vi "subVI_read_write_ADC_DAC.vi"(7 "CH":bool[](array[boolean])=[FALSE, FALSE, TRUE, FALSE, FALSE, TRUE, FALSE, FALSE, FALSE, FALSE, FALSE, FALSE, FALSE, FALSE, FALSE, FALSE], 8 "DAC2":bool[](array[boolean]), 9 "DAC1":bool[](array[boolean]), 10 "error in":errorcluster, 11 "FPGA VI Reference In":refnum<k20>) -> (0 "FPGA VI Reference Out":refnum<k20>, 1 "i":dbl, 2 "GAIN":i16, 3 "UNI":i16, 4 "error out":errorcluster)   [LabVIEW 2018]
uses:
  <vilib>/Utility/error.llb/Error Cluster From Error Code.vi
  <vilib>/rvi/errors/niLvFpgaAdjustHostInterfaceError.vi
  <vilib>/rvi/interface/nirviReadWriteControl/nirviReadWriteControl.xnode
  NiFpgaLv.dll
  <vilib>/rvi/interface/Simulation/niFpgaSimulationCallBeginRW.vi
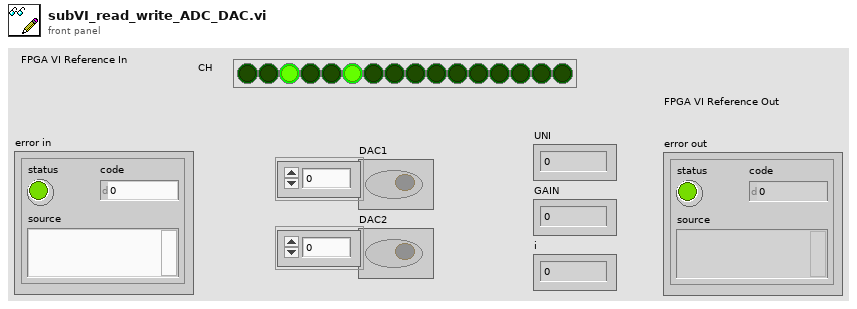
[diagram p1: front panel]
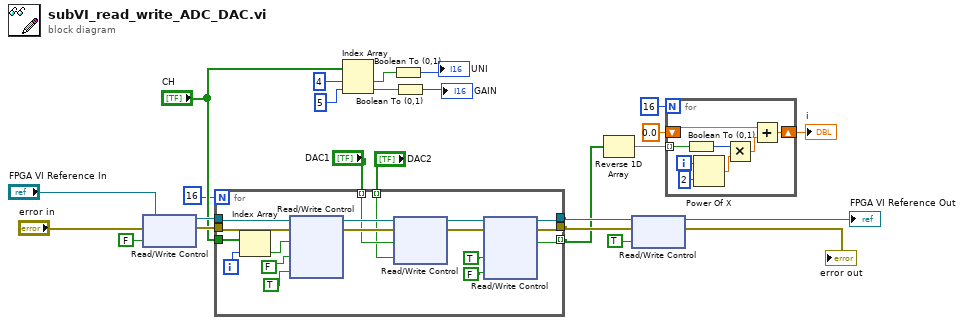
[diagram p0: block diagram]
diagram:
  n1 = xnode "Read/Write Control"("FPGA VI Reference In"="FPGA VI Reference In", "error in"="error in", "CS"=FALSE) -> ("FPGA VI Reference Out"=w13:refnum<k20>, "error out"=w12:errorcluster)
  n2 = for {
    N: 16 -> [_]
    tunnel: w13 -> [w34]
    tunnel: w12 -> [w33]
    tunnel: [w28] -> w14 mode=indexing
    tunnel: [w27] -> w16
    tunnel: [w26] -> w15
    tunnel: "CH" -> [w32]
    tunnel: "DAC1" -> [w30] mode=indexing
    tunnel: "DAC2" -> [w29] mode=indexing
    i -> [w31]
    n3 = Index Array(array=w32, index=w31) -> (element=w43:bool)
    n4 = xnode "Read/Write Control"("FPGA VI Reference In"=w34, "error in"=w33, "MOSI1"=w43, "CLK2"=FALSE ("CLK"), "CLK1"=TRUE ("CLK")) -> ("FPGA VI Reference Out"=w40:refnum<k20>, "error out"=w39:errorcluster)
    n5 = xnode "Read/Write Control"("FPGA VI Reference In"=w40, "error in"=w39, "MOSI2"=w30, "MOSI3"=w29) -> ("FPGA VI Reference Out"=w38:refnum<k20>, "error out"=w37:errorcluster)
    n6 = xnode "Read/Write Control"("FPGA VI Reference In"=w38, "error in"=w37, "CLK2"=TRUE, "CLK1"=FALSE) -> ("FPGA VI Reference Out"=w27:refnum<k20>, "error out"=w26:errorcluster, "MISO1"=w28:bool)
  }
  n7 = Index Array(array="CH", index #1=4 ("index"), index #2=5 ("index")) -> (element #1=w18:bool, element #2=w17:bool)
  n8 = Boolean To (0,1)(Boolean=w18) -> (0, 1=→"UNI":i16)
  n9 = Boolean To (0,1)(Boolean=w17) -> (0, 1=→"GAIN":i16)
  n10 = Reverse 1D Array(array=w14) -> (reversed array=w23:bool[])
  n11 = xnode "Read/Write Control"("FPGA VI Reference In"=w16, "error in"=w15, "CS"=TRUE) -> ("FPGA VI Reference Out"=→"FPGA VI Reference Out":refnum<k20>, "error out"=→"error out":errorcluster)
  n12 = for {
    N: 16 -> [_]
    shift-right: [w49] -> w5
    shift-left: 0.0 -> [w50]
    tunnel: w23 -> [w44] mode=indexing
    i -> [w45]
    n13 = Boolean To (0,1)(Boolean=w44) -> (0, 1=w51:i16)
    n14 = Power Of X(1:2 ("y"), 2:w45) -> (0:w47:dbl)
    n15 = Multiply(x=w51, y=w47) -> (x*y=w48:dbl)
    n16 = Add(x=w50, y=w48) -> (x+y=w49:dbl)
  }
  "i" <- w5
